vi "Line Profile.vi"() -> ()   [LabVIEW 2014]
doc: "Use this template to build a VI to use as a subVI."
uses:
  <vilib>/vision/NI_Vision_Development_Module.lvlib
panel:
  out "Line Profile":cluster{"x0":sgl, "dx":sgl, "Pixels Line":sgl[]}(graph)
  out "Src":T1(plugin-control)
  # ":: MVi Framework V1.0 ::\nAuthor:Gaoke Yang\nEmail: gaoke.yang@yahoo.com\nWeb: www.mvicontrol.com\nCopyright (C) 2015, MVI Technologies All Rights Reserved"
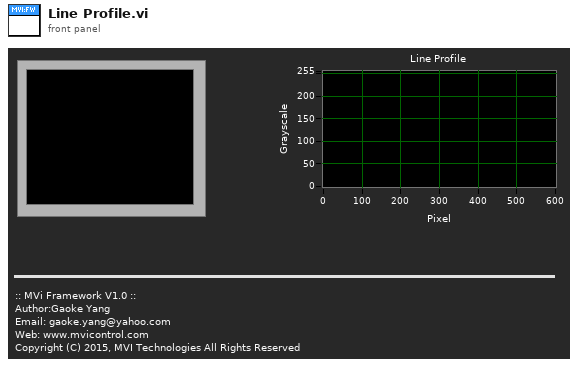
[diagram p1: front panel]
types:
  T1 = typedef "IMAQ Image.ctl" = refnum<image>
  T2 = typedef "Image Type" = u32
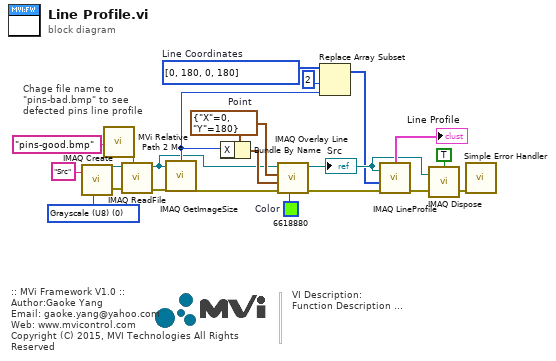
[diagram p0: block diagram]
diagram:
  w5 = i32[] [0, 180, 0, 180]  # Line Coordinates
  w11 = u32 6618880  # Color
  w7 = cluster{"X":i32, "Y":i32} {"X"=0, "Y"=180}  # Point
  w16 = T2 0 items=["Grayscale (U8)", "Grayscale (I16)", "Grayscale (SGL)", "Complex (CSG)", "RGB (U32)", "HSL (U32)", "RGB (U64)", "Grayscale (U16)"] ("Image Type")
  # "Chage file name to \n\"pins-bad.bmp\" to see\ndefected pins line profile"
  # "VI Description:\nFunction Description ..."
  # ":: MVi Framework V1.0 ::\nAuthor:Gaoke Yang\nEmail: gaoke.yang@yahoo.com\nWeb: www.mvicontrol.com\nCopyright (C) 2015, MVI Technologies All Rights Reserved"
  n1 = call "IMAQ Create"("Image Name"="Src" ("name or relative path"), "Image Type"=w16) -> ("New Image"=w17:T1, "error out"=w15:errorcluster)  [unwired: 2 in, 1 out]
  n2 = call "MVi Relative Path 2 Me.vi"("Relative Path"="pins-good.bmp" ("name or relative path")) -> ("Appended Dir"=w18:path)  [unwired: 5 in, 1 out]
  n3 = call "IMAQ ReadFile"("File Path"=w18, "error in (no error)"=w15, "Image"=w17) -> ("error out"=w9:errorcluster, "Image Out"=w1:T1)  [unwired: 4 in, 3 out]
  n4 = call "IMAQ GetImageSize"("Image"=w1, "error in (no error)"=w9) -> ("X Resolution"=w3:i32, "error out"=w8:errorcluster)  [unwired: 2 in, 1 out]
  n5 = Bundle By Name(cluster=w7, "X"=w3) -> (w6:cluster{"X":i32, "Y":i32})
  n6 = call "IMAQ Overlay Line"("Color"=w11, "error in (no error)"=w8, "End Point"=w6, "Start Point"=w7, "Image"=w1) -> ("error out"=w12:errorcluster, "Image Out"=w10:T1)  [unwired: 5 in]
  "Src" <- w10
  n7 = Replace Array Subset(array=w5, new element=w3, index=2) -> (w2:i32[])
  n8 = call "IMAQ LineProfile"("error in (no error)"=w12, "Line Coordinates"=w2, "Image"=w10) -> ("error out"=w14:errorcluster, "Line Graph"=→"Line Profile":cluster{"x0":sgl, "dx":sgl, "Pixels Line":sgl[]})  [unwired: 2 in, 2 out]
  n9 = call "IMAQ Dispose"("All Images? (No)"=TRUE, "Image"=w10, "error in (no error)"=w14) -> ("error out"=w19:errorcluster)  [unwired: 3 out]
  n10 = call <vilib>:"Simple Error Handler.vi"("error in (no error)"=w19) -> ()  [unwired: 1 in, 8 out]
